vi "GCOMM Set Path.vi"(8 "error in":errorcluster, 10 "path":string, 11 "session in":T1) -> (0 "error out":errorcluster, 3 "session out":T1)   [LabVIEW 2020]
doc: "Sets path of the generic COM port multiplexer."
uses:
  GCOMM Session.ctl
  GCOMM Signal.ctl
  GCOMM Virtual Channel.ctl
  GCOMM Logic State.ctl
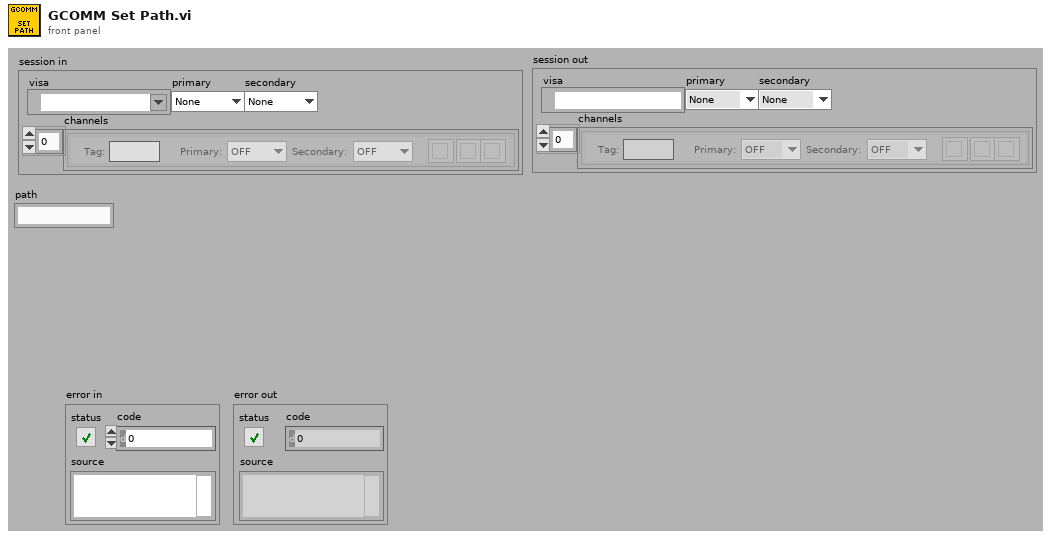
[diagram p1: front panel]
types:
  T1 = typedef "GCOMM Session.ctl" = cluster{"visa":refnum<visa-resource-name>, "primary":T2, "secondary":T2, "channels":T3[]}
  T2 = typedef "GCOMM Signal.ctl" = enum16{"None", "DTR", "RTS"}
  T3 = typedef "GCOMM Virtual Channel.ctl" = cluster{"Primary:":T4, "Secondary:":T4, "btn clr":bool, "btn up":bool, "btn down":bool, "Tag:":string}
  T4 = typedef "GCOMM Logic State.ctl" = enum16{"OFF", "ON"}
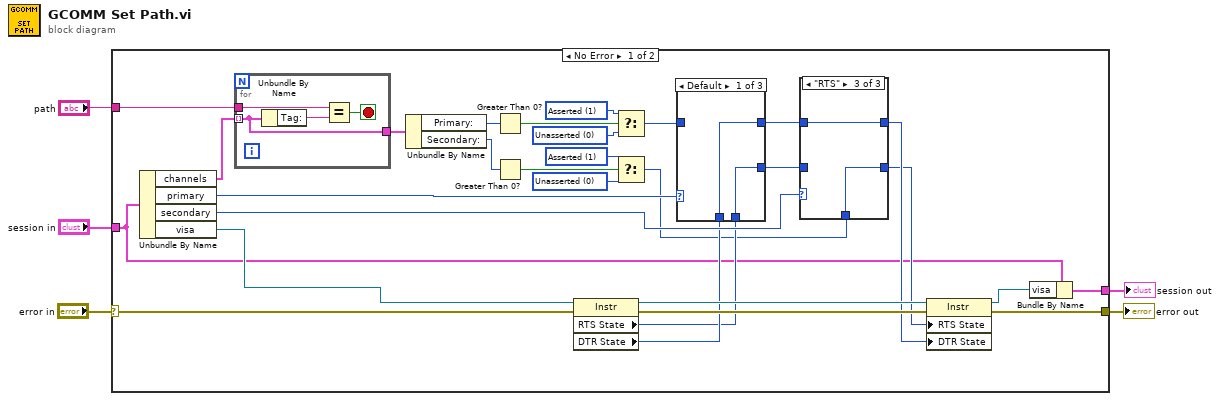
[diagram p0: block diagram]
diagram:
  n1 = case shown="No Error" "error in" {
    selector: "error in" -> [w20 w52]
    tunnel: [w34 w52] -> w5
    tunnel: "session in" -> [w8 w51]
    tunnel: [w6 w51] -> w3
    tunnel: "path" -> [w32 _]
    frame No Error {
      w24 = i16 0 items=["Unknown"=-1, "Unasserted"=0, "Asserted"=1] ("Serial Settings:Modem Line Settings:Line RTS State")
      w25 = i16 1 items=["Unknown"=-1, "Unasserted"=0, "Asserted"=1] ("Serial Settings:Modem Line Settings:Line RTS State")
      w27 = i16 0 items=["Unknown"=-1, "Unasserted"=0, "Asserted"=1] ("Serial Settings:Modem Line Settings:Line RTS State")
      w28 = i16 1 items=["Unknown"=-1, "Unasserted"=0, "Asserted"=1] ("Serial Settings:Modem Line Settings:Line RTS State")
      n2 = Unbundle By Name(w8) -> ("channels"=w33:T3[], "primary"=w30:T2, "secondary"=w16:T2, "visa"=w18:refnum<visa-resource-name>)
      n3 = for {
        tunnel: w33 -> [w47] mode=indexing
        tunnel: w32 -> [w49]
        tunnel: [w47] -> w31
        stop <- w48 stop-if-true
        n4 = Unbundle By Name(w47) -> ("Tag:"=w50:string)
        n5 = Equal?(x=w49, y=w50) -> (x = y?=w48:bool)
      }
      n6 = Unbundle By Name(w31) -> ("Primary:"=w29:T4, "Secondary:"=w23:T4)
      n7 = Greater Than 0?(x=w29) -> (x > 0?=w26:bool)
      n8 = Greater Than 0?(x=w23) -> (x > 0?=w22:bool)
      n9 = property class="Instr"(reference=w18, error in=w20) -> (reference out=w17:refnum<visa-resource-name>, error out=w19:errorcluster, "RTS State"=w14:i16, "DTR State"=w15:i16)
      n10 = Select(t=w28, s=w26, f=w27) -> (s? t:f=w21:i16)
      n11 = Select(t=w25, s=w22, f=w24) -> (s? t:f=w11:i16)
      n12 = case shown="Default" w30 {
        tunnel: w21 -> [_ w44 w46]
        tunnel: [w42 w44 w45] -> w13
        tunnel: w15 -> [w42 _ w45]
        tunnel: [w41 w43 w46] -> w12
        tunnel: w14 -> [w41 w43 _]
        frame Default {
        }
        frame "DTR" {
        }
        frame "RTS" {
        }
      }
      n13 = case shown="\"RTS\"" w16 {
        tunnel: w13 -> [w36 _ w40]
        tunnel: [w36 w38 w40] -> w10
        tunnel: [w35 w37 w39] -> w9
        tunnel: w12 -> [w35 w37 _]
        tunnel: w11 -> [_ w38 w39]
        frame Default {
        }
        frame "DTR" {
        }
        frame "RTS" {
        }
      }
      n14 = property class="Instr"(reference=w17, error in=w19, "RTS State"=w9, "DTR State"=w10) -> (reference out=w7:refnum<visa-resource-name>, error out=w34:errorcluster)
      n15 = Bundle By Name(cluster=w8, "visa"=w7) -> (w6:T1)
    }
    frame Error {
    }
  }
  "error out" <- w5
  "session out" <- w3
